vi "oscilloscope.vi"() -> ()   [LabVIEW 2024]
doc: "This example shows how to configure multiple channels and acquire waveforms from multiple channels."
uses:
  <instrlib>/_Template - Scope/Template - Scope.lvlib
  <instrlib>/_Template - Scope/Public/Data/Read Waveform (Multiple).vi
panel:
  out "error in":errorcluster
  in  "Multiwaveform Acquisition Enabled (OFF)":bool
  out "output array":dbl[](array[numeric])
  out "VISA resource name out":refnum<visa-resource-name>
  out "error out":errorcluster
  in  "Vertical offset D":dbl
  in  "Vertical range D":dbl
  in  "Probe Attenuation D (10.0)":dbl=10.0
  in  "Vertical Coupling D (1: DC)":u16(ring)=1 items=["AC", "DC", "Ground"]
  in  "Vertical offset C":dbl
  in  "Vertical range C":dbl
  in  "Probe Attenuation C (10.0)":dbl=10.0
  in  "Vertical Coupling C (1: DC)":u16(ring)=1 items=["AC", "DC", "Ground"]
  in  "Vertical offset B":dbl
  in  "Vertical range B":dbl
  in  "Probe Attenuation B (10.0)":dbl=10.0
  in  "Vertical Coupling B":u16(ring)=1 items=["AC", "DC", "Ground"]
  out "Waveform Data":dbl[](array[numeric]) caption="Waveform Array" format="%^.3e"
  out "Starting point (1)":i32=1 caption="Waveform (1)"
  in  "Trigger Level (0.0 V)":dbl
  in  "Trigger Slope (0: Rising)":u16(ring) items=["Rising", "Falling"]
  in  "Vertical offset A":dbl
  in  "Vertical range A":dbl
  in  "Maximum Time (10000 ms)":u32=10000
  in  "Probe Attenuation A (10.0)":dbl=10.0
  in  "Vertical Coupling A":u16(ring)=1 items=["AC", "DC", "Ground"]
  out "Waveform Data":waveform(dbl)[](graph)
  in  "VISA resource name":refnum<visa-resource-name>
  # "Channel A"
  # "Channel B"
  # "Channel C"
  # "Channel D"
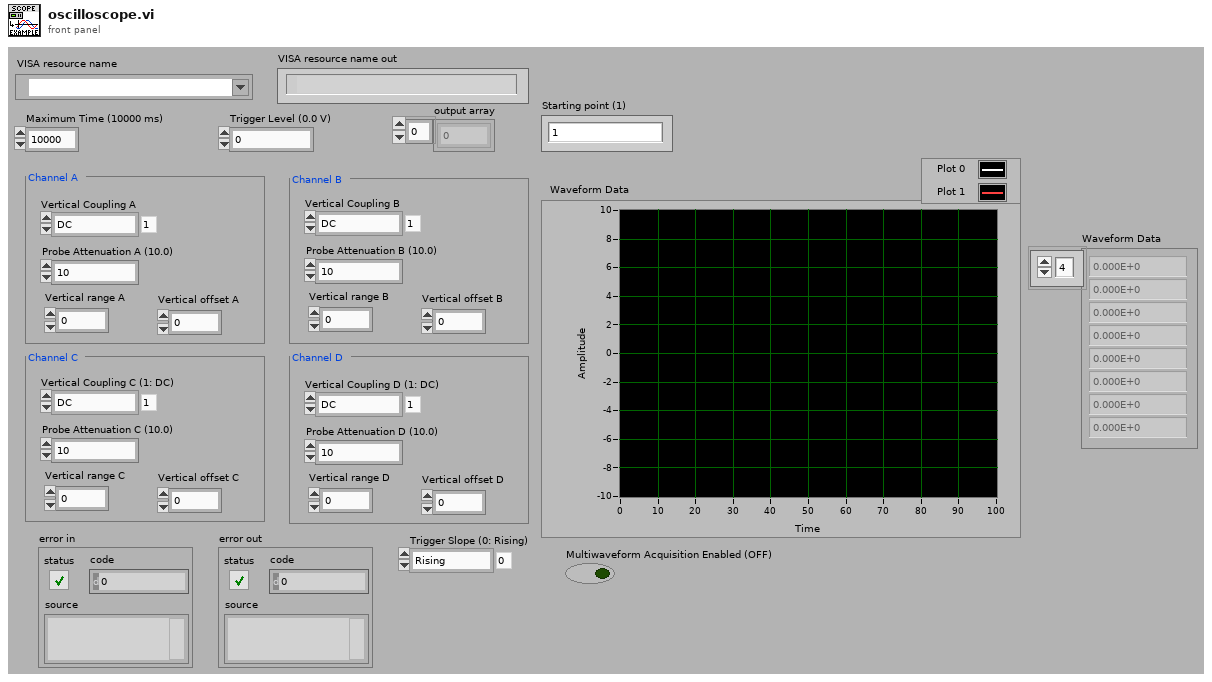
[diagram p1: front panel]
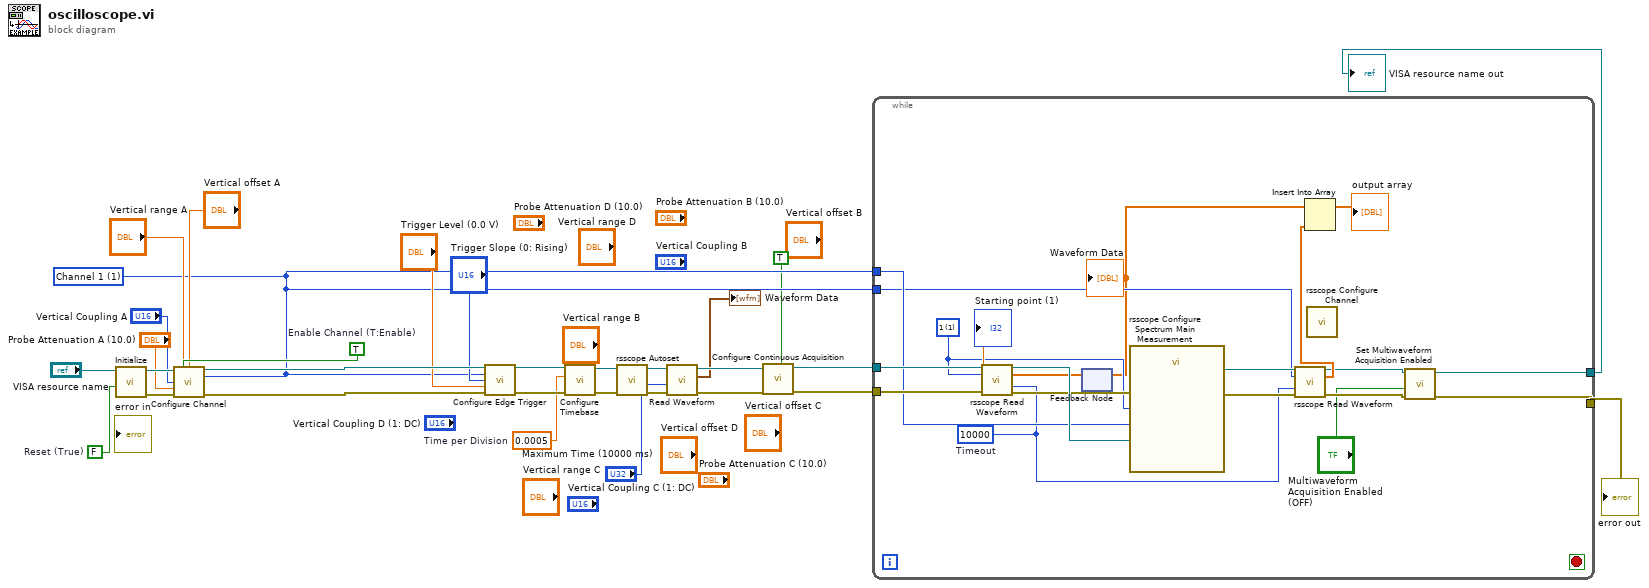
[diagram p0: block diagram]
diagram:
  w9 = u16 1 items=["Channel 1"=1, "Channel 2"=2, "Channel 3"=3, "Channel 4"=4] ("Channel (1: Channel 1)")
  w18 = TRUE  # Enable Channel (T:Enable)
  w19 = FALSE  # Reset (True)
  w24 = 0.0005  # Time per Division
  n1 = call <instrlib>:"Initialize.vi"("Reset (True)"=w19, "VISA resource name"="VISA resource name") -> ("error out"=w29:errorcluster, "VISA resource name out"=w30:refnum<visa-resource-name>)  [unwired: 8 in]
  n2 = call <instrlib>:"Configure Channel.vi"("VISA resource name"=w30, "Enable Channel (T:Enable)"=w18, "Channel (1: Channel 1)"=w9, "Vertical Coupling (1: DC)"="Vertical Coupling A", "Probe Attenuation (1.0)"="Probe Attenuation A (10.0)", "error in (no error)"=w29, "Vertical Range (10.0 V)"="Vertical range A", "Vertical Offset (0.0 V)"="Vertical offset A") -> ("VISA resource name out"=w26:refnum<visa-resource-name>, "error out"=w25:errorcluster)  [unwired: 6 in]
  n3 = call <instrlib>:"Configure Edge Trigger.vi"("VISA resource name"=w26, "Trigger Source (1: Channel 1)"=w9, "Trigger Slope (0: Rising)"="Trigger Slope (0: Rising)", "Trigger Level (0.0 V)"="Trigger Level (0.0 V)", "error in (no error)"=w25) -> ("VISA resource name out"=w28:refnum<visa-resource-name>, "error out"=w27:errorcluster)  [unwired: 9 in]
  n4 = call <instrlib>:"Configure Timebase.vi"("error in (no error)"=w27, "Time per Division (0.0005 s)"=w24, "VISA resource name"=w28) -> ("error out"=w7:errorcluster, "VISA resource name out"=w6:refnum<visa-resource-name>)  [unwired: 7 in]
  n5 = call <instrlib>:"rsscope Autoset.vi"("error in (no error)"=w7, "VISA resource name"=w6) -> ("error out"=w4:errorcluster, "VISA resource name out"=w5:refnum<visa-resource-name>)  [unwired: 8 in]
  n6 = call-poly <instrlib>:"Read Waveform.vi"("error in (no error)"=w4, "Maximum Time (10000 ms)"="Maximum Time (10000 ms)", "VISA resource name"=w5) -> ("error out"=w21:errorcluster, "Waveform Data"=→"Waveform Data":waveform(dbl)[], "VISA resource name out"=w23:refnum<visa-resource-name>)  [unwired: 6 in]
  n7 = call <instrlib>:"Configure Continuous Acquisition.vi"("error in (no error)"=w21, "Enable Continuous Acquisition (T:Enable)"=TRUE, "VISA resource name"=w23) -> ("error out"=w10:errorcluster, "VISA resource name out"=w3:refnum<visa-resource-name>)  [unwired: 7 in]
  n8 = while {
    tunnel: w3 -> [w50]
    tunnel: w10 -> [w49]
    tunnel: w9 -> [w45]
    tunnel: w9 -> [w41]
    tunnel: [w32] -> w2
    tunnel: [w31] -> w1
    stop <- _ stop-if-true
    w44 = 1 items=["1"=1, "2"=2, "3"=3, "4"=4] ("Channel (1)")
    w40 = 10000  # Timeout
    n9 = call <instrlib>:"rsscope Read Waveform.vi"("VISA resource name"=w50, "Channel (1)"=w44, "Maximum Time (5000)"=w40, "error in (no error)"=w49) -> ("VISA resource name out"=w47:refnum<visa-resource-name>, "Waveform Array"=w39:dbl[], "Initial X"=→"Starting point (1)":dbl, "error out"=w46:errorcluster)  [unwired: 7 in, 1 out]
    n10 = feedback-in #1(w39) -> ()
    n11 = feedback #1() -> (w38:dbl[])  [unwired: 1 in]
    "Waveform Data" <- w38
    n12 = call <instrlib>:"rsscope Configure Spectrum Main Measurement.vi"("Measurement Function (Channel Power)"=w45, "error in (no error)"=w46, "Measurement (1)"=w44, "VISA resource name"=w47) -> ("error out"=w42:errorcluster, "VISA resource name out"=w43:refnum<visa-resource-name>)  [unwired: 6 in]
    n13 = call <instrlib>:"rsscope Read Waveform.vi"("VISA resource name"=w43, "Channel (1)"=w41, "Maximum Time (5000)"=w40, "error in (no error)"=w42) -> ("VISA resource name out"=w35:refnum<visa-resource-name>, "Waveform Array"=w36:dbl[], "error out"=w34:errorcluster)  [unwired: 7 in, 2 out]
    n14 = Insert Into Array(array=w38, new element=w36) -> (→"output array":dbl[])  [unwired: 1 in]
    n15 = call <instrlib>:"rsscope Configure Channel.vi"() -> ()  [unwired: 10 in, 2 out]
    n16 = call "Set Multiwaveform Acquisition Enabled"("error in (no error)"=w34, "Multiwaveform Acquisition Enabled (OFF)"="Multiwaveform Acquisition Enabled (OFF)", "instrument handle"=w35) -> ("error out"=w32:errorcluster, "instrument handle out"=w31:refnum<visa-resource-name>)  [unwired: 7 in]
  }
  "error out" <- w2
  "VISA resource name out" <- w1
